vi "Handle SpecPage Project Name Change.vi"(9 "Project Name New Value":string, 10 "Project Name Old Value":string, 11 "Project Root in":path) -> (3 "Project Root out":path)   [LabVIEW 2016]
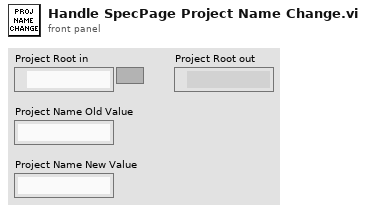
[diagram p1: front panel]
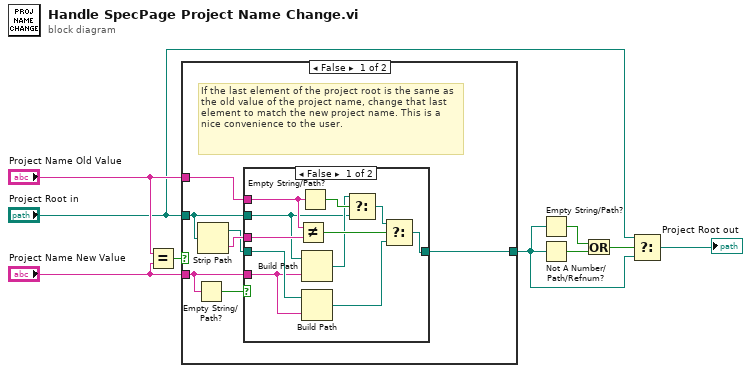
[diagram p0: block diagram]
diagram:
  n1 = Equal?(x="Project Name Old Value", y="Project Name New Value") -> (x = y?=w9:bool)
  n2 = case shown="False" w9 {
    tunnel: "Project Root in" -> [w15 w29]
    tunnel: [w14 w29] -> w3
    tunnel: "Project Name Old Value" -> [w11 _]
    tunnel: "Project Name New Value" -> [w10 _]
    frame False {
      # "If the last element of the project root is the same as the old value of the project name, change that last element to match the new project name. This is a nice convenience to the user."
      n3 = Empty String/Path?(string/path=w10) -> (empty?=w12:bool)
      n4 = Strip Path(path=w15) -> (stripped path=w13:path, name=w16:string)
      n5 = case shown="False" w12 {
        tunnel: w16 -> [w27 _]
        tunnel: w11 -> [w23 _]
        tunnel: w15 -> [w18 _]
        tunnel: [w26 w28] -> w14
        tunnel: w13 -> [w25 w28]
        tunnel: w10 -> [w17 _]
        frame False {
          n6 = Not Equal?(x=w23, y=w27) -> (x != y?=w22:bool)
          n7 = Empty String/Path?(string/path=w23) -> (empty?=w21:bool)
          n8 = Build Path(base path=w18, name or relative path=w17) -> (appended path=w19:path)
          n9 = Build Path(base path=w25, name or relative path=w17) -> (appended path=w24:path)
          n10 = Select(t=w19, s=w21, f=w18) -> (s? t:f=w20:path)
          n11 = Select(t=w20, s=w22, f=w24) -> (s? t:f=w26:path)
        }
        frame True {
        }
      }
    }
    frame True {
    }
  }
  n12 = Empty String/Path?(string/path=w3) -> (empty?=w5:bool)
  n13 = Not A Number/Path/Refnum?(number/path/refnum=w3) -> (NaN/Path/Refnum?=w6:bool)
  n14 = Or(x=w5, y=w6) -> (x .or. y?=w4:bool)
  n15 = Select(t="Project Root in", s=w4, f=w3) -> (s? t:f=→"Project Root out":path)
